vi "parse_LinkState.vi"(8 "error in":errorcluster, 11 "msg in":string) -> (0 "error out":errorcluster, 2 "LinkState":T1, 3 "msg out":string)   [LabVIEW 2012]
uses:
  <userlib>/ROSforLV/ROS/parsing/std_msgs/subs/parse_string_scalar.vi
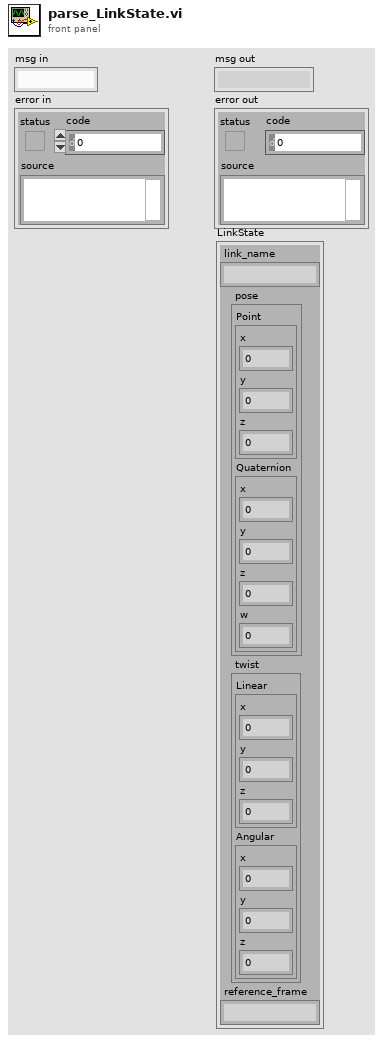
[diagram p1: front panel]
types:
  T1 = cluster{" link_name":string, " pose":cluster{"Point":cluster{"x":dbl, "y":dbl, "z":dbl}, "Quaternion":cluster{"x":dbl, "y":dbl, "z":dbl, "w":dbl}}, " twist":cluster{"Linear":cluster{"x":dbl, "y":dbl, "z":dbl}, "Angular":cluster{"x":dbl, "y":dbl, "z":dbl}}, " reference_frame":string}
  T2 = cluster{"Point":cluster{"x":dbl, "y":dbl, "z":dbl}, "Quaternion":cluster{"x":dbl, "y":dbl, "z":dbl, "w":dbl}}
  T3 = cluster{"Linear":cluster{"x":dbl, "y":dbl, "z":dbl}, "Angular":cluster{"x":dbl, "y":dbl, "z":dbl}}
  T4 = cluster{"string":string, "Pose":cluster{"Point":cluster{"x":dbl, "y":dbl, "z":dbl}, "Quaternion":cluster{"x":dbl, "y":dbl, "z":dbl, "w":dbl}}, "Twist":cluster{"Linear":cluster{"x":dbl, "y":dbl, "z":dbl}, "Angular":cluster{"x":dbl, "y":dbl, "z":dbl}}, "string":string}
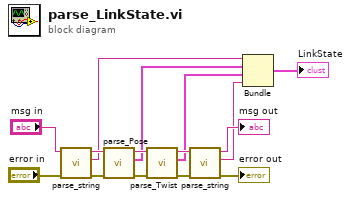
[diagram p0: block diagram]
diagram:
  n1 = call-poly <userlib>:"parse_string.vi"("error in"="error in", "msg in"="msg in") -> ("error out"=w12:errorcluster, "string"=w5:string, "msg out"=w13:string)  [unwired: 3 in]
  n2 = call <userlib>:"parse_Pose.vi"("error in"=w12, "msg in"=w13) -> ("error out"=w10:errorcluster, "Pose"=w4:T2, "msg out"=w11:string)  [unwired: 3 in]
  n3 = call <userlib>:"parse_Twist.vi"("error in"=w10, "msg in"=w11) -> ("error out"=w8:errorcluster, "Twist"=w3:T3, "msg out"=w9:string)  [unwired: 3 in]
  n4 = call-poly <userlib>:"parse_string.vi"("error in"=w8, "msg in"=w9) -> ("error out"=→"error out":errorcluster, "string"=w2:string, "msg out"=→"msg out":string)  [unwired: 3 in]
  n5 = Bundle("string"=w5, "Pose"=w4, "Twist"=w3, "string"=w2) -> (→"LinkState":T4)  [unwired: 1 in]
